vi "WaveGraph_Initiation.vi"(3 "Container State":T4 caption="容器状态", 4 "Previous State":variant caption="前期状态", 5 "Previous Version":T3 caption="前期版本") -> (2 "Current State":T1={"图例拖动State"=FALSE, "统计图例拖动State"=FALSE, "峰值图例拖动State"=FALSE, "图例拖动坐标 队列"=refnum, "统计图例拖动坐标 队列"=refnum, "峰值图例拖动坐标 队列"=refnum, "后台服务VI 引用"=refnum, "控件引用簇 队列"=refnum, "User Event"=refnum, "属性簇"={"曲线条数"=0, "曲线属性簇数组"=[], "文本属性簇数组"=[], "信息属性簇"={"图例"=FALSE, "信息_统计量"=FALSE, "信息_统计量_有效值"=FALSE, "信息_统计量_最大值"=FALSE, "信息_统计量_最小值"=FALSE, "信息_统计量_峰峰值"=FALSE, "信息_统计量_均值"=FALSE, "信息_统计量_方差"=FALSE, "信息_统计量_所有通道"=FALSE, "光标列表"=0, "数量"=1.0, "排列"=0, "格式"=0, "精度"=3.0}}} caption="当前状态" {"属性簇"."信息属性簇"."格式" items=["十进制", "科学值"]; "属性簇"."信息属性簇"."排列" items=["幅值"]; "属性簇"."信息属性簇"."光标列表" items=["单光标", "双光标", "峰值光标"]; "属性簇"."曲线属性簇数组"."曲线_填充基线" items=["无", "零", "负无穷大", "正无穷大"]; "属性簇"."曲线属性簇数组"."曲线_线条宽度" items=["0", "1", "2", "3", "4", "5"]; "属性簇"."曲线属性簇数组"."曲线_线条样式" items=["实线", "粗虚线", "细虚线", "点划线", "双点划线"]})   [LabVIEW 2012, in "WaveGraphX.xctl"]
uses:
  WaveGraphX.xctl
  WaveGraph_State.ctl
  <resource>/importtools/Common/Event/NISAST Event.lvclass
  <vilib>/Utility/miscctls.llb/LVPoint32TypeDef.ctl
  GraphStates.ctl
  <vilib>/_xctls/Container State.ctl
  <vilib>/_xctls/Version.ctl
  <vilib>/_xctls/XControlSupport.lvlib
panel:
  in  "Default Indicator State":T1={"图例拖动State"=FALSE, "统计图例拖动State"=FALSE, "峰值图例拖动State"=FALSE, "图例拖动坐标 队列"=refnum, "统计图例拖动坐标 队列"=refnum, "峰值图例拖动坐标 队列"=refnum, "后台服务VI 引用"=refnum, "控件引用簇 队列"=refnum, "User Event"=refnum, "属性簇"={"曲线条数"=0, "曲线属性簇数组"=[], "文本属性簇数组"=[], "信息属性簇"={"图例"=FALSE, "信息_统计量"=FALSE, "信息_统计量_有效值"=FALSE, "信息_统计量_最大值"=FALSE, "信息_统计量_最小值"=FALSE, "信息_统计量_峰峰值"=FALSE, "信息_统计量_均值"=FALSE, "信息_统计量_方差"=FALSE, "信息_统计量_所有通道"=FALSE, "光标列表"=0, "数量"=1.0, "排列"=0, "格式"=0, "精度"=3.0}}} caption="默认显示控件状态" {"属性簇"."信息属性簇"."格式" items=["十进制", "科学值"]; "属性簇"."信息属性簇"."排列" items=["幅值"]; "属性簇"."信息属性簇"."光标列表" items=["单光标", "双光标", "峰值光标"]; "属性簇"."曲线属性簇数组"."曲线_填充基线" items=["无", "零", "负无穷大", "正无穷大"]; "属性簇"."曲线属性簇数组"."曲线_线条宽度" items=["0", "1", "2", "3", "4", "5"]; "属性簇"."曲线属性簇数组"."曲线_线条样式" items=["实线", "粗虚线", "细虚线", "点划线", "双点划线"]}
  in  "Default Control State":T1={"图例拖动State"=FALSE, "统计图例拖动State"=FALSE, "峰值图例拖动State"=FALSE, "图例拖动坐标 队列"=refnum, "统计图例拖动坐标 队列"=refnum, "峰值图例拖动坐标 队列"=refnum, "后台服务VI 引用"=refnum, "控件引用簇 队列"=refnum, "User Event"=refnum, "属性簇"={"曲线条数"=0, "曲线属性簇数组"=[], "文本属性簇数组"=[], "信息属性簇"={"图例"=FALSE, "信息_统计量"=FALSE, "信息_统计量_有效值"=FALSE, "信息_统计量_最大值"=FALSE, "信息_统计量_最小值"=FALSE, "信息_统计量_峰峰值"=FALSE, "信息_统计量_均值"=FALSE, "信息_统计量_方差"=FALSE, "信息_统计量_所有通道"=FALSE, "光标列表"=0, "数量"=1.0, "排列"=0, "格式"=0, "精度"=3.0}}} caption="默认输入控件状态" {"属性簇"."信息属性簇"."格式" items=["十进制", "科学值"]; "属性簇"."信息属性簇"."排列" items=["幅值"]; "属性簇"."信息属性簇"."光标列表" items=["单光标", "双光标", "峰值光标"]; "属性簇"."曲线属性簇数组"."曲线_填充基线" items=["无", "零", "负无穷大", "正无穷大"]; "属性簇"."曲线属性簇数组"."曲线_线条宽度" items=["0", "1", "2", "3", "4", "5"]; "属性簇"."曲线属性簇数组"."曲线_线条样式" items=["实线", "粗虚线", "细虚线", "点划线", "双点划线"]}
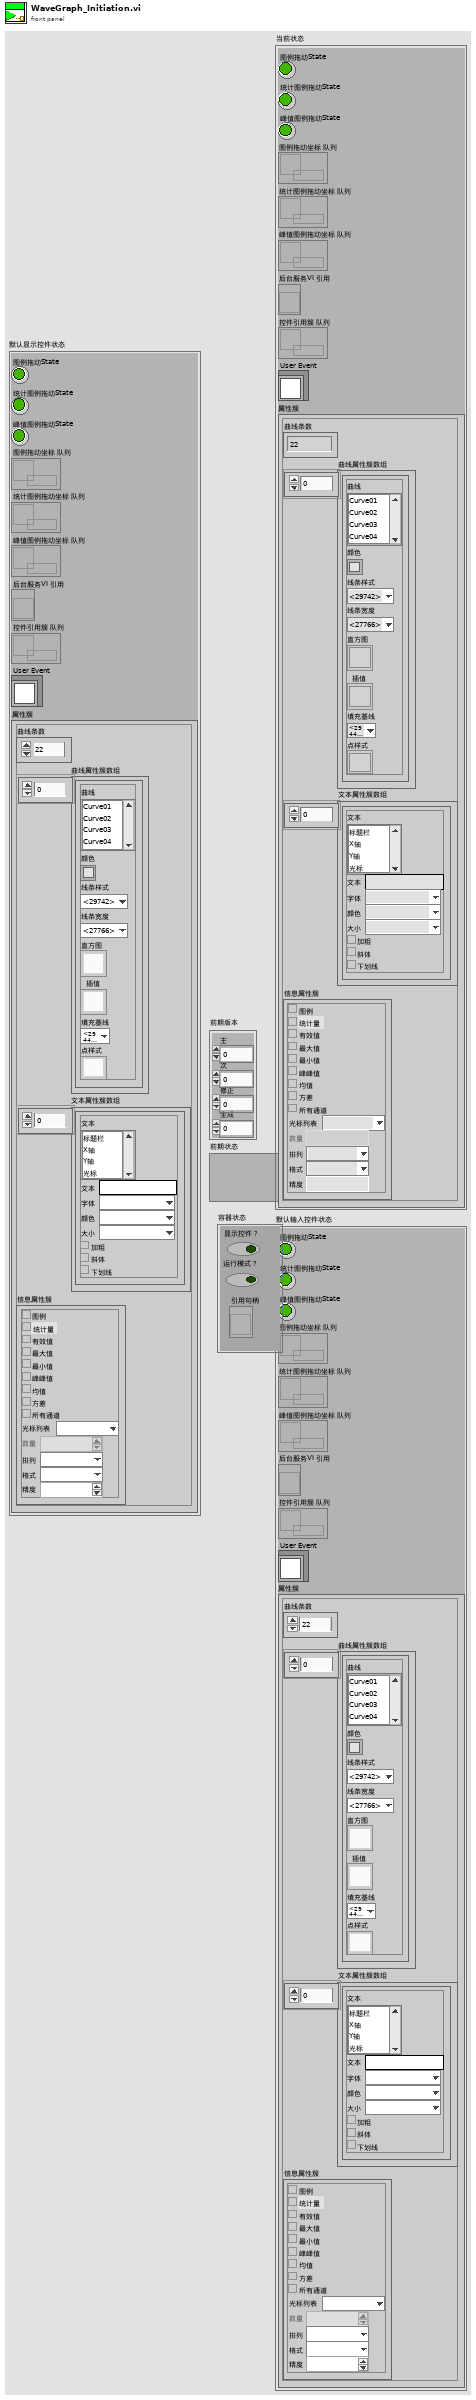
[diagram p1: front panel]
types:
  T1 = typedef "WaveGraphX.xctl/WaveGraph_State.ctl" = cluster{"图例拖动State":bool, "统计图例拖动State":bool, "峰值图例拖动State":bool, "图例拖动坐标 队列":refnum<queue>, "统计图例拖动坐标 队列":refnum<queue>, "峰值图例拖动坐标 队列":refnum<queue>, "后台服务VI 引用":refnum<vi>, "控件引用簇 队列":refnum<queue>, "User Event":refnum<class "NISAST Event.lvclass">, "属性簇":T2}
  T2 = typedef "WaveGraphX.xctl/GraphStates.ctl" = cluster{"曲线条数":u8, "曲线属性簇数组":cluster{"曲线_曲线":i32, "曲线_颜色":u32, "曲线_线条样式":u16, "曲线_线条宽度":u16, "曲线_直方图":u16, "曲线_插值":u16, "曲线_填充基线":u16, "曲线_点样式":u16}[], "文本属性簇数组":cluster{"文本_文本":i32, "文本":string, "字体":u16, "颜色":u16, "大小":u16, "加粗":bool, "斜体":bool, "下划线":bool}[], "信息属性簇":cluster{"图例":bool, "信息_统计量":bool, "信息_统计量_有效值":bool, "信息_统计量_最大值":bool, "信息_统计量_最小值":bool, "信息_统计量_峰峰值":bool, "信息_统计量_均值":bool, "信息_统计量_方差":bool, "信息_统计量_所有通道":bool, "光标列表":u16, "数量":dbl, "排列":u16, "格式":u16, "精度":dbl}}
  T3 = typedef "XControlSupport.lvlib/Version.ctl" = cluster{"Major":u16, "Minor":u16, "Fix":u16, "Build":u16}
  T4 = typedef "XControlSupport.lvlib/Container State.ctl" = cluster{"Indicator?":bool, "Run Mode?":bool, " Refnum":refnum<vi>}
  T5 = typedef "LVPoint32TypeDef.ctl" = cluster{"Horizontal":i32, "Vertical":i32}
  T6 = cluster{"图例拖动State":refnum<vi>, "统计图例拖动State":refnum<vi>, "峰值图例拖动State":refnum<vi>, "图例":refnum<vi>, "统计图例":refnum<vi>, "峰值图例":refnum<vi>}
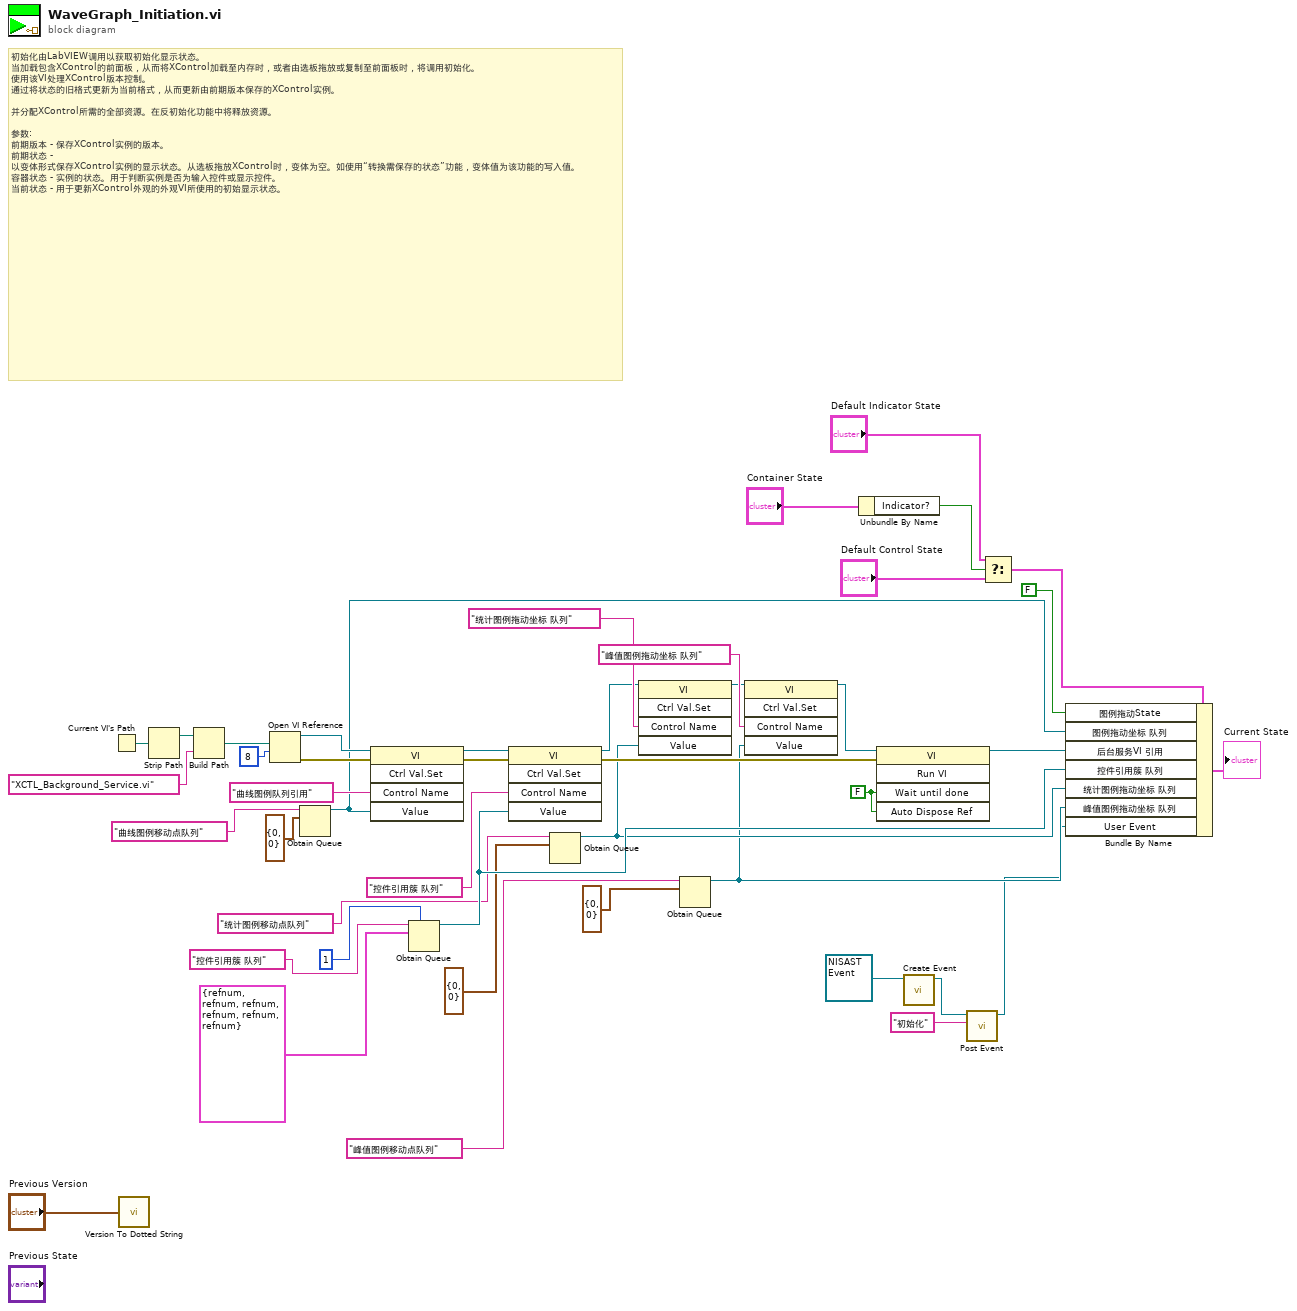
[diagram p0: block diagram]
diagram:
  w30 = FALSE ("自动销毁引用")
  # "初始化由LabVIEW调用以获取初始化显示状态。\n当加载包含XControl的前面板，从而将XControl加载至内存时，或者由选板拖放或复制至前面板时，将调用初始化。\n使用该VI处理XControl版本控制。\n通过将状态的旧格式更新为当前格式，从而更新由前期版本保存的XControl实例。\n\n并分配XControl所需的全部资源。在反初始化功能中将释放资源。\n\n参数: \n前期版本 - 保存XControl实例的版本。\n前期状态 - 以变体形式保存XControl实例的显示状态。从选板拖放XControl时，变体为空。如使用“转换需保存的状态”功能，变体值为该功能的写入值。\n容器状态 - 实例的状态。用于判断实例是否为输入控件或显示控件。\n当前状态 - 用于更新XControl外观的外观VI所使用的初始显示状态。"
  n1 = Current VI's Path() -> (path=w39:path)
  n2 = call <vilib>:"Version To Dotted String.vi"("Version"="Previous Version") -> ()  [unwired: 1 out]
  n3 = Strip Path(path=w39) -> (stripped path=w38:path)  [unwired: 1 out]
  n4 = Build Path(base path=w38, name or relative path="XCTL_Background_Service.vi" ("名称或相对路径")) -> (appended path=w36:path)
  n5 = Open VI Reference(vi path=w36, options=8 ("选项")) -> (vi reference=w34:refnum<vi>, error out=w29:errorcluster)  [unwired: 4 in]
  n6 = Obtain Queue(name (unnamed)="曲线图例移动点队列" ("名称（未命名）"), element data type=T5 {"Horizontal"=0, "Vertical"=0} ("坐标")) -> (queue out=w26:refnum<queue>)  [unwired: 3 in, 2 out]
  n7 = invoke class="VI" method="Ctrl Val.Set"(reference=w34, error in=w29, "Control Name"="曲线图例队列引用" ("控件名"), "Value"=w26) -> (reference out=w18:refnum<vi>, error out=w16:errorcluster)  [unwired: 1 in, 3 out]
  n8 = Obtain Queue(max queue size (-1, unlimited)=1 ("队列最大值（-1，无限）"), name (unnamed)="控件引用簇 队列" ("名称（未命名）"), element data type=T6 {"图例拖动State"=refnum, "统计图例拖动State"=refnum, "峰值图例拖动State"=refnum, "图例"=refnum, "统计图例"=refnum, "峰值图例"=refnum} ("输出簇")) -> (queue out=w20:refnum<queue>)  [unwired: 2 in, 2 out]
  n9 = invoke class="VI" method="Ctrl Val.Set"(reference=w18, error in=w16, "Control Name"="控件引用簇 队列" ("控件名"), "Value"=w20) -> (reference out=w8:refnum<vi>, error out=w17:errorcluster)  [unwired: 1 in, 3 out]
  n10 = Obtain Queue(name (unnamed)="统计图例移动点队列" ("名称（未命名）"), element data type=T5 {"Horizontal"=0, "Vertical"=0} ("坐标")) -> (queue out=w6:refnum<queue>)  [unwired: 3 in, 2 out]
  n11 = invoke class="VI" method="Ctrl Val.Set"(reference=w8, "Control Name"="统计图例拖动坐标 队列" ("控件名"), "Value"=w6) -> (reference out=w9:refnum<vi>)  [unwired: 2 in, 4 out]
  n12 = Obtain Queue(name (unnamed)="峰值图例移动点队列" ("名称（未命名）"), element data type=T5 {"Horizontal"=0, "Vertical"=0} ("坐标")) -> (queue out=w5:refnum<queue>)  [unwired: 3 in, 2 out]
  n13 = invoke class="VI" method="Ctrl Val.Set"(reference=w9, "Control Name"="峰值图例拖动坐标 队列" ("控件名"), "Value"=w5) -> (reference out=w7:refnum<vi>)  [unwired: 2 in, 4 out]
  n14 = Unbundle By Name("Container State") -> ("Indicator?"=w41:bool)
  n15 = invoke class="VI" method="Run VI"(reference=w7, error in=w17, "Wait until done"=w30, "Auto Dispose Ref"=w30) -> (reference out=w24:refnum<vi>)  [unwired: 1 in, 4 out]
  n16 = call-dynamic "Create Event.vi"("Event in"=refnum<class "NISAST Event.lvclass"> refnum ("NISAST Event.lvclass")) -> ("Event out"=w3:refnum<class "NISAST Event.lvclass">)  [unwired: 8 in, 2 out]
  n17 = call-dynamic "Post Event.vi"("Event Name"="初始化", "Event in"=w3) -> ("Event out"=w1:refnum<class "NISAST Event.lvclass">)  [unwired: 8 in, 1 out]
  n18 = Select(t="Default Indicator State", s=w41, f="Default Control State") -> (s? t:f=w27:T1)
  n19 = Bundle By Name(cluster=w27, "图例拖动State"=FALSE, "图例拖动坐标 队列"=w26, "后台服务VI 引用"=w24, "控件引用簇 队列"=w20, "统计图例拖动坐标 队列"=w6, "峰值图例拖动坐标 队列"=w5, "User Event"=w1) -> (→"Current State":T1)
